vi "Launch Root Panel Window.vi"(5 "Window Position (Maximize First Call)":refnum<class "Window Position.lvclass">, 6 "timeout in ms (-1)":i32=-1, 7 "Autoshow? (T)":bool=TRUE, 8 "Error In":errorcluster, 10 "Title":string, 11 "Panel Actor in":refnum<class "Panel Actor.lvclass">) -> (0 "Error Out":errorcluster, 2 "Actor's Enqueuer":refnum<class "Message Enqueuer.lvclass">)   [LabVIEW 2017, in "MGI-Panel Actor.lvlib"]
doc: "Launches a Root Panel using the window Panel type.\n\n<B>Panel Actor In:</B> Panel Actor object to launch\n<B>Title:</B> Sets the default title for the window.\n<B>Autoshow?</B> If Autoshow? is TRUE, then the Window will be displayed on initialization. If it is FALSE, then the Show method must be called manually.\n<B>Window Position:</B> Window Position object to control window position behavior.\n<B>timeout in ms</B> Time to wait for the panel to initialize\n<B>Error In:</B> Describes error conditions that occur before this node runs.\n\n<B>Actor's Enqueuer:</B> Enqueuer for newly spawned actor\n<B>Error Out:</B> Contains error information.\n----\nCopyright: MGI 2018\nAuthor: Derek Trepanier"
uses:
  MGI-Panel Actor.lvlib
  Panel Actor/Panel Actor.lvclass
  panel-manager/Source/Window Position/Window Position.lvclass
  <vilib>/ActorFramework/Message Enqueuer/Message Enqueuer.lvclass
  panel-manager/Source/Window Position/Maximize/Maximize.lvclass
  D:/software/LabView_PanelManager/panel-manager/Source/Window Position/Window Position.lvclass
  panel-manager/Source/Panel/Window/Window.lvclass
  D:/software/LabView_PanelManager/panel-manager/Source/Panel/Panel.lvclass
  panel-manager/Source/Panel/Window/Window.vi
  panel-manager/Source/MGI-Panel Manager.lvlib
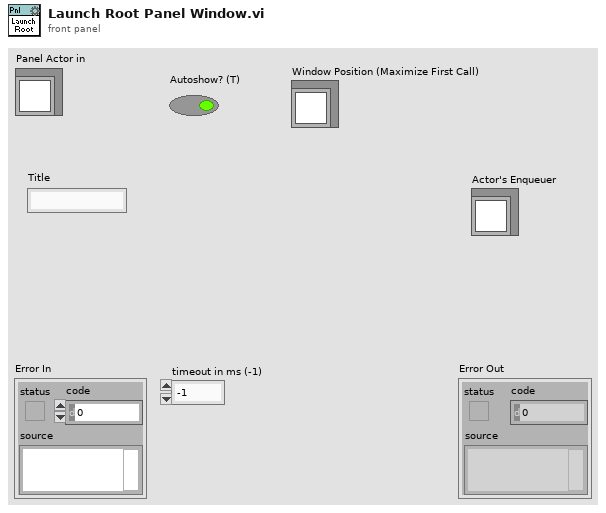
[diagram p1: front panel]
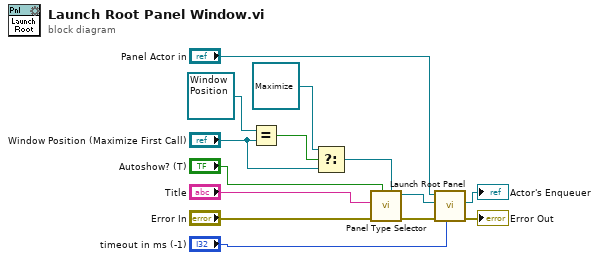
[diagram p0: block diagram]
diagram:
  n1 = Equal?(x=refnum<class "Window Position.lvclass"> refnum ("y"), y="Window Position (Maximize First Call)") -> (x = y?=w2:bool)
  n2 = Select(t=refnum<class "Maximize.lvclass"> refnum ("MGI-Panel Manager.lvlib:Maximize.lvclass"), s=w2, f="Window Position (Maximize First Call)") -> (s? t:f=w4:refnum<class "Window Position.lvclass">)
  n3 = call-poly "Panel Type Selector.vi"("Window Position"=w4, "Autoshow? (T)"="Autoshow? (T)", "error in (no error)"="Error In", "Default Title"="Title") -> ("error out"=w7:errorcluster, "Window out"=w8:refnum<class "Window.lvclass">)  [unwired: 6 in]
  n4 = call "Launch Root Panel.vi"("timeout in ms (-1)"="timeout in ms (-1)", "Error In"=w7, "Panel"=w8, "Panel Actor in"="Panel Actor in") -> ("Error Out"=→"Error Out":errorcluster, "Actor's Enqueuer"=→"Actor's Enqueuer":refnum<class "Message Enqueuer.lvclass">)  [unwired: 6 in]
